vi "WriteObj.vi"(0 "reference in":refnum<class "Logger.lvclass">, 5 "device":T1, 11 "error in (no error)":errorcluster) -> (4 "reference out":refnum<class "Logger.lvclass">, 15 "error out":errorcluster)   [LabVIEW 2019, in "Logger.lvclass"]
uses:
  Logger.lvclass
  ObjData.ctl
  ObjType.ctl
  Logger.lvclass/Logger.ctl
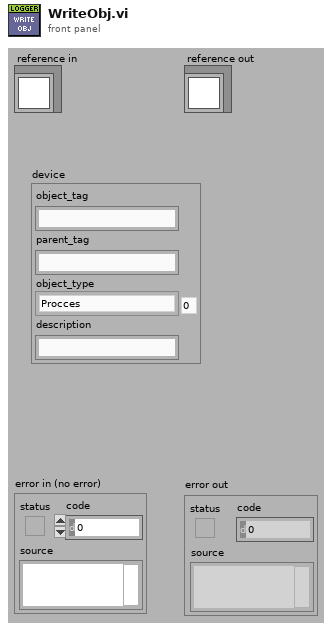
[diagram p1: front panel]
types:
  T1 = typedef "Logger.lvclass/ObjData.ctl" = cluster{"object_tag":string, "parent_tag":string, "object_type":T2, "description":string}
  T2 = typedef "Logger.lvclass/ObjType.ctl" = enum16{"Procces", "Device", "SignalA", "SignalD", "DI", "DO", "DA", "AI", "AO", "AA", "GUI"}
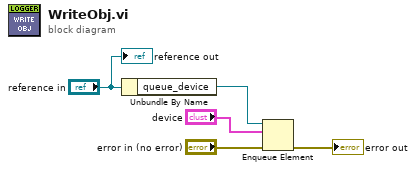
[diagram p0: block diagram]
diagram:
  n1 = Unbundle By Name("reference in") -> ("queue_device"=w1:refnum<queue>)
  n2 = Enqueue Element(queue=w1, element="device", error in (no error)="error in (no error)") -> (error out=→"error out":errorcluster)  [unwired: 1 in, 2 out]
  "reference out" <- "reference in"
